vi "欧姆龙PLC通讯Fans UDP-写PLC寄存器编码-输入数据为U8.vi"(10 "数据U8":u8[](array[numeric]), 11 "起始地址16":string) -> (3 "写入数据编码":string)   [LabVIEW 2014]
panel:
  out "数据U8   2":u8[](array[numeric])
  out "16bit寄存器个数":string
  out "字符串":string
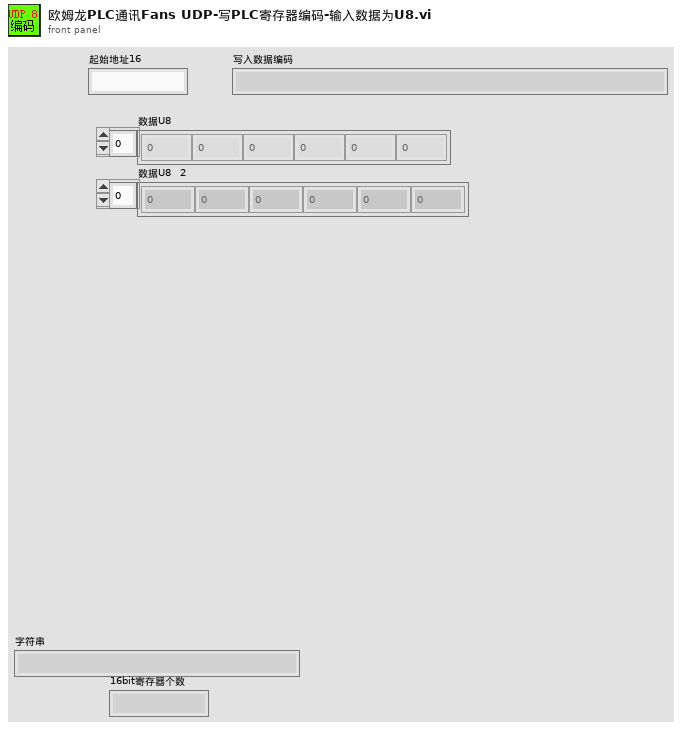
[diagram p1: front panel]
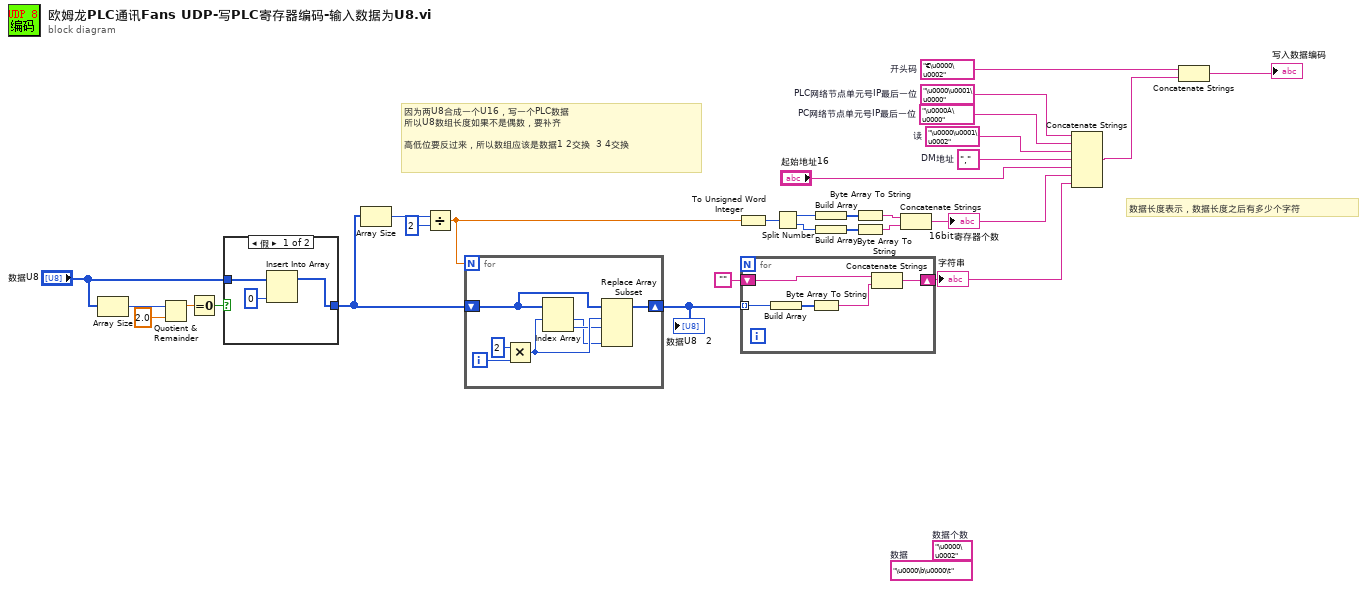
[diagram p0: block diagram]
diagram:
  w26 = "\u0000À\u0000"  # PC网络节点单元号IP最后一位
  w25 = "\u0000\u0001\u0000"  # PLC网络节点单元号IP最后一位
  w24 = "€\u0000\u0002"  # 开头码
  (unwired) "\u0000\b\u0000\t"  # 数据
  (unwired) "\u0000\u0002"  # 数据个数
  w22 = "‚"  # DM地址
  w21 = "\u0000\u0001\u0002"  # 读
  # "因为两U8合成一个U16，写一个PLC数据\n所以U8数组长度如果不是偶数，要补齐\n\n高低位要反过来，所以数组应该是数据1 2交换  3 4交换"
  # "数据长度表示，数据长度之后有多少个字符"
  n1 = Array Size(array="数据U8") -> (size(s)=w7:i32)
  n2 = Quotient & Remainder(x=w7, y=2.0) -> (x-y*floor(x/y)=w6:dbl)  [unwired: 1 out]
  n3 = Equal To 0?(x=w6) -> (x = 0?=w4:bool)
  n4 = case shown="假" w4 {
    tunnel: "数据U8" -> [w31 w32]
    tunnel: [w30 w32] -> w2
    frame False {
      n5 = Insert Into Array(array=w31, new element=u8 0 ("新元素/子数组")) -> (w30:u8[])  [unwired: 1 in]
    }
    frame True {
    }
  }
  n6 = Array Size(array=w2) -> (size(s)=w12:i32)
  n7 = Divide(x=w12, y=2) -> (x/y=w3:dbl)
  n8 = for {
    N: w3 -> [_]
    shift-right: [w35] -> w1
    shift-left: w2 -> [w36]
    i -> [w39]
    n9 = Multiply(x=2, y=w39) -> (x*y=w37:i32)
    n10 = Index Array(array=w36, index #1=w37) -> (element #1=w33:u8, element #2=w34:u8)  [unwired: 1 in]
    n11 = Replace Array Subset(array=w36, new element #1=w34, index #1=w37, new element #2=w33) -> (w35:u8[])  [unwired: 1 in]
  }
  "数据U8   2" <- w1
  n12 = To Unsigned Word Integer(number=w3) -> (unsigned 16bit integer=w13:u16)
  n13 = for {
    tunnel: w1 -> [w41] mode=indexing
    shift-right: [w43] -> w10
    shift-left: "" -> [w44]
    n14 = Build Array(w41) -> (w40:u8[])
    n15 = Byte Array To String(unsigned byte array=w40) -> (string=w42:string)
    n16 = Concatenate Strings(w44, w42) -> (w43:string)
  }
  "字符串" <- w10
  n17 = Split Number(x=w13) -> (hi(x)=w14:u8, lo(x)=w15:u8)
  n18 = Build Array(w14) -> (w16:u8[])
  n19 = Build Array(w15) -> (w17:u8[])
  n20 = Byte Array To String(unsigned byte array=w16) -> (string=w18:string)
  n21 = Byte Array To String(unsigned byte array=w17) -> (string=w19:string)
  n22 = Concatenate Strings(w18, w19) -> (w9:string)
  "16bit寄存器个数" <- w9
  n23 = Concatenate Strings(w25, w26, w21, w22, "起始地址16", w9, w10) -> (w27:string)
  n24 = Concatenate Strings(w24, w27) -> (→"写入数据编码":string)
